vi "BRig_Host__Loop_Producer__tcp_System__Data_prepareFilepaths_target.vi"(8 "input_arrFilenames":string[](array[string]), 9 "input_nFilenames":i32, 10 "input_storagePath":string, 11 "input_expPrefix":string) -> (1 "output_arrPath_target":path[](array[path]))   [LabVIEW 2014]
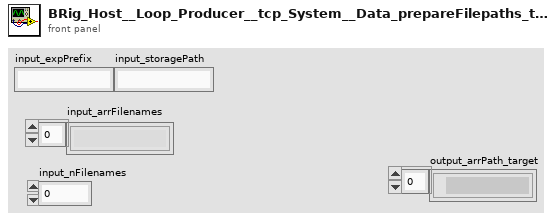
[diagram p1: front panel]
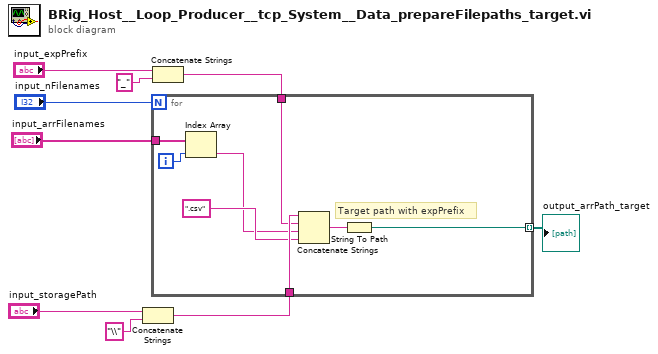
[diagram p0: block diagram]
diagram:
  n1 = Concatenate Strings("input_storagePath", "\\" ("string")) -> (w2:string)
  n2 = Concatenate Strings("input_expPrefix", "_" ("string")) -> (w6:string)
  n3 = for {
    N: "input_nFilenames" -> [_]
    tunnel: w6 -> [w13]
    tunnel: "input_arrFilenames" -> [w17]
    tunnel: w2 -> [w14]
    tunnel: [w10] -> w1 mode=indexing
    i -> [w16]
    # "Target path with expPrefix"
    n4 = Index Array(array=w17, index=w16) -> (element=w11:string)
    n5 = Concatenate Strings(w14, w13, w11, ".csv" ("string")) -> (w15:string)
    n6 = String To Path(string=w15) -> (path=w10:path)
  }
  "output_arrPath_target" <- w1
